vi "time_string_to_time_stamp.vi"(11 "Array in":string[](array[string])) -> (3 "Array out":timestamp[](array[timestamp]))   [LabVIEW 2017]
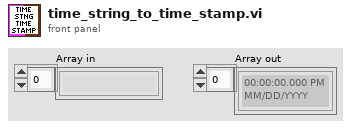
[diagram p1: front panel]
types:
  T1 = typedef "LVDateTimeRec.ctl" = cluster{"fractional second":dbl, "second":i32, "minute":i32, "hour":i32, "day of month":i32, "month":i32, "year":i32, "day of week":i32, "day of year":i32, "DST":i32}
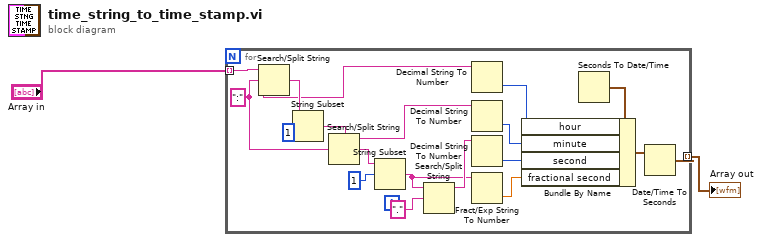
[diagram p0: block diagram]
diagram:
  n1 = for {
    tunnel: "Array in" -> [w11] mode=indexing
    tunnel: [w19] -> w1 mode=indexing
    w18 = ":" ("format string")
    n2 = Search/Split String(string=w11, search string/char (-)=w18) -> (substring before match=w7:string, match + rest of string=w16:string)  [unwired: 1 in, 1 out]
    n3 = String Subset(string=w16, offset (0)=1) -> (substring=w15:string)  [unwired: 1 in]
    n4 = Search/Split String(string=w15, search string/char (-)=w18) -> (substring before match=w6:string, match + rest of string=w13:string)  [unwired: 1 in, 1 out]
    n5 = String Subset(string=w13, offset (0)=1) -> (substring=w5:string)  [unwired: 1 in]
    n6 = Search/Split String(string=w5, search string/char (-)="." ("format string")) -> (substring before match=w10:string)  [unwired: 1 in, 2 out]
    n7 = Decimal String To Number(string=w7) -> (number=w8:i32)  [unwired: 2 in, 1 out]
    n8 = Decimal String To Number(string=w6) -> (number=w9:i32)  [unwired: 2 in, 1 out]
    n9 = Decimal String To Number(string=w10) -> (number=w3:i32)  [unwired: 2 in, 1 out]
    n10 = Fract/Exp String To Number(string=w5) -> (number=w4:dbl)  [unwired: 3 in, 1 out]
    n11 = Seconds To Date/Time() -> (date time rec=w20:T1)  [unwired: 2 in]
    n12 = Bundle By Name(cluster=w20, "hour"=w8, "minute"=w9, "second"=w3, "fractional second"=w4) -> (w21:T1)
    n13 = Date/Time To Seconds(2:w21) -> (0:w19:timestamp)  [unwired: 1 in]
  }
  "Array out" <- w1
